vi "Compound Interest.vi"() -> ()   [LabVIEW 2021]
panel:
  in  "Compunded":u16(ring) items=["yearly"=1, "half yearly"=2, "quarterly"=4, "monthly"=12, "bi-weekly"=26, "weekly"=52, "daily"=109]
  in  "Annual Interest Rate(%)":dbl
  in  "Finished":bool
  in  "Calculate":bool
  out "Amount($)":dbl
  in  "Principal":dbl
  in  "Years":dbl
  # "Compound Interest Calculator"
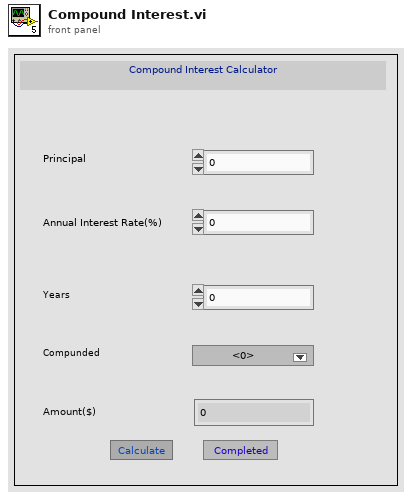
[diagram p1: front panel]
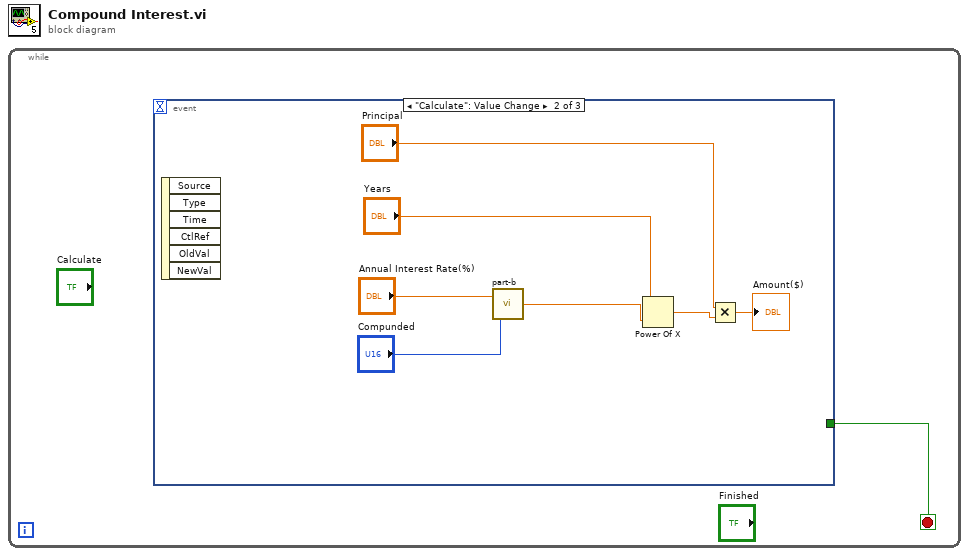
[diagram p0: block diagram]
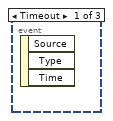
[diagram p2: hidden frame]
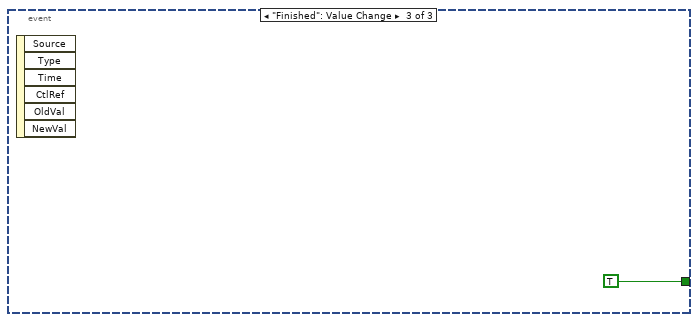
[diagram p3: hidden frame]
diagram:
  n1 = while {
    stop <- w1 stop-if-true
    n2 = event shown="[1] \"Calculate\": Value Change" {
      selector: _ -> [_ _ _]
      dyn-events: _ -> [_ _ _]
      timeout: _ -> [_ _ _]
      tunnel: [_ _ TRUE] -> w1
      event Timeout {
        n3 = event-data() -> ()  [unwired: 1 in, 3 out]
      }
      event "Calculate": Value Change {
        n4 = event-data() -> ()  [unwired: 1 in, 6 out]
        n5 = call "part-b.vi"("Compunded"="Compunded", "Annual Interest Rate(%)"="Annual Interest Rate(%)") -> ("Rate of Y1"=w2:dbl)
        n6 = Power Of X(1:w2, 2:"Years") -> (0:w7:dbl)
        n7 = Multiply(x="Principal", y=w7) -> (x*y=→"Amount($)":dbl)
      }
      event "Finished": Value Change {
        n8 = event-data() -> ()  [unwired: 1 in, 6 out]
      }
    }
  }
